vi "Client Connect To URL Test.vi"() -> ()   [LabVIEW 2014, in "ESP8266 WiFi Wrapper.lvlib"]
uses:
  <vilib>/Aledyne-TSXperts/Arduino Compatible Compiler for LabVIEW/addons/ESP8266 WiFi Wrapper/ESP8266 WiFi Wrapper.lvlib
panel:
  out "Connected?":bool
  in  "Port":u16=80
  in  "URL address":string="www.helloworld.com"
  out "Error Out":errorcluster
  in  "Error In":errorcluster
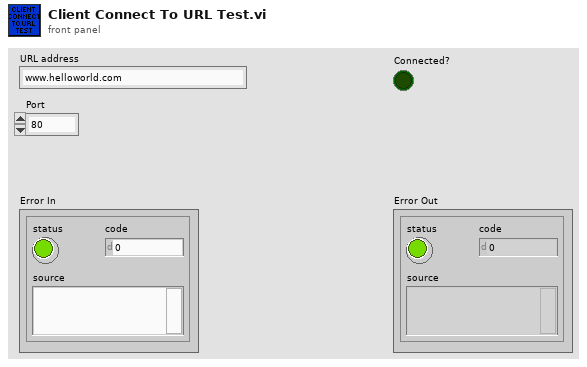
[diagram p1: front panel]
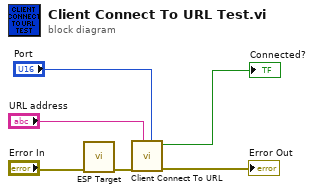
[diagram p0: block diagram]
diagram:
  n1 = call <vilib>:"ESP Target.vi"("Error In"="Error In") -> ("Error Out"=w2:errorcluster)  [unwired: 10 in]
  n2 = call <vilib>:"Client Connect To URL.vi"("Port"="Port", "URL address"="URL address", "Error In"=w2) -> ("Error Out"=→"Error Out":errorcluster, "Connected?"=→"Connected?":bool)  [unwired: 7 in]
